vi "get_trigger_type.vi"(8 "error in (no error)":errorcluster, 10 "call chain":string[](array[string])=["GenericToplevelComponent.lvclass:send_generic_trigger.vi", "GenericStage.lvclass:send_trigger.vi", "StageDL090409Scaffold.lvclass:run.vi", "GenericToplevelComponent.lvclass:manager.vi:1", "GenericStage.lvclass:test_generic.vi"], 11 "GenericToplevelComponent in":refnum<class "GenericToplevelComponent.lvclass">) -> (0 "error out":errorcluster, 1 "TLC type out":T1=enum."ImagingMode", 2 "found?":bool, 3 "GenericToplevelComponent out":refnum<class "GenericToplevelComponent.lvclass">, 4 "component found class":string, 5 "type of component found string":string)   [LabVIEW 2010, in "GenericToplevelComponent.lvclass"]
uses:
  GenericToplevelComponent.lvclass
  enumerations/top-level_component_type_enum.ctl
panel:
  in  "TLC type":T1=enum."ImagingMode"
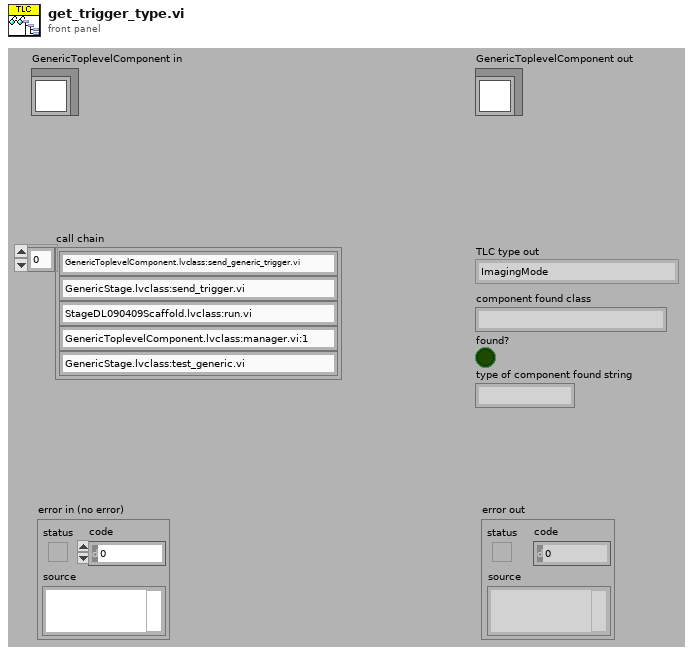
[diagram p1: front panel]
types:
  T1 = typedef "top-level_component_type_enum.ctl" = enum16{"undefined", "ImagingMode", "ScanHead", "DAQ", "ImageAssembler", "Display", "DataCollection", "Analyser", "Stimulator", "ExperimentController", "Instrument", "Stage"}
  T2 = enum16{"undefined", "ImagingMode", "ScanHead", "DAQ", "ImageAssembler", "Display", "DataCollection", "Analyser", "Stimulator", "ExperimentController", "Instrument", "Stage"}
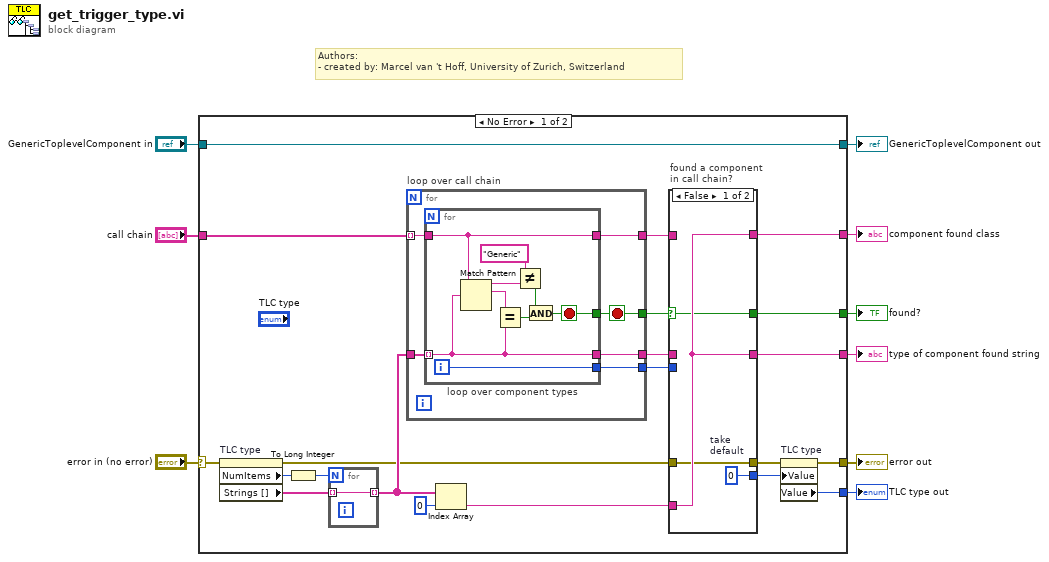
[diagram p0: block diagram]
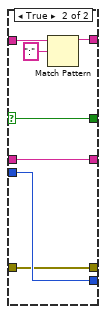
[diagram p2: hidden frame]
diagram:
  # "Authors: \n- created by: Marcel van 't Hoff, University of Zurich, Switzerland"
  n1 = case shown="No Error" "error in (no error)" {
    selector: "error in (no error)" -> [w14 w59]
    tunnel: [w29 _] -> w2
    tunnel: [w27 _] -> w4
    tunnel: [w21 _] -> w3
    tunnel: [w16 w59] -> w7
    tunnel: "call chain" -> [w19 _]
    tunnel: "GenericToplevelComponent in" -> [w18 w58]
    tunnel: [w18 w58] -> w5
    tunnel: [w15 _] -> w1
    frame No Error {
      n2 = property on="TLC type" class="Enum (strict)"(error in=w14) -> (error out=w13:errorcluster, "NumItems"=w12:u32, "Strings []"=w11:string[])  [unwired: 1 in, 1 out]
      n3 = To Long Integer(number=w12) -> (32bit integer=w30:i32)
      n4 = for {
        N: w30 -> [_]
        tunnel: w11 -> [w57] mode=indexing
        tunnel: [w57] -> w23 mode=indexing
      }
      n5 = for "loop over call chain" {
        tunnel: w19 -> [w46] mode=indexing
        tunnel: w23 -> [w47]
        tunnel: [w45] -> w28
        tunnel: [w44] -> w26
        tunnel: [w43] -> w25
        tunnel: [w42] -> w20
        stop <- w43 stop-if-true
        n6 = for "loop over component types" {
          tunnel: w47 -> [w50] mode=indexing
          tunnel: w46 -> [w49]
          tunnel: [w51] -> w43
          tunnel: [w50] -> w45
          tunnel: [w49] -> w44
          tunnel: [w48] -> w42
          i -> [w48]
          stop <- w51 stop-if-true
          n7 = Match Pattern(string=w49, regular expression=w50) -> (before substring=w53:string, match substring=w52:string)  [unwired: 1 in, 2 out]
          n8 = Equal?(x=w52, y=w50) -> (x = y?=w56:bool)
          n9 = Not Equal?(x="Generic" ("before substring"), y=w53) -> (x != y?=w55:bool)
          n10 = And(x=w55, y=w56) -> (x .and. y?=w51:bool)
        }
      }
      n11 = Index Array(array=w23, index=0) -> (element=w24:string)
      n12 = case "found a component\nin call chain?" shown="False" w25 {
        selector: w25 -> [w33 w40]
        tunnel: [w34 w41] -> w29
        tunnel: w28 -> [_ w41]
        tunnel: [w34 w37] -> w27
        tunnel: w26 -> [_ w38]
        tunnel: w24 -> [w34 _]
        tunnel: [w33 w40] -> w21
        tunnel: w20 -> [_ w36]
        tunnel: [w32 w36] -> w10
        tunnel: [w31 w35] -> w17
        tunnel: w13 -> [w31 w35]
        frame False {
          w32 = 0  # take  default
        }
        frame True {
          n13 = Match Pattern(string=w38, regular expression=":") -> (before substring=w37:string)  [unwired: 1 in, 3 out]
        }
      }
      n14 = property on="TLC type" class="Enum (strict)"(error in=w17, "Value"=w10) -> (error out=w16:errorcluster, "Value"=w15:T2)  [unwired: 1 in, 1 out]
    }
    frame Error {
    }
  }
  "error out" <- w7
  "GenericToplevelComponent out" <- w5
  "component found class" <- w4
  "found?" <- w3
  "type of component found string" <- w2
  "TLC type out" <- w1
